vi "CloseEthernetIP connection.vi"(8 "error in (no error)":errorcluster, 11 ".NET Refnum in":refnum<k24>) -> (0 "error out":errorcluster)   [LabVIEW 2022 SP3, in "Motor Controller.lvclass"]
uses:
  Motor Controller.lvclass
  C:/projects/Digilens_IPLC/Classes/Motor Controller/EEIP.dll
  EEIP.dll
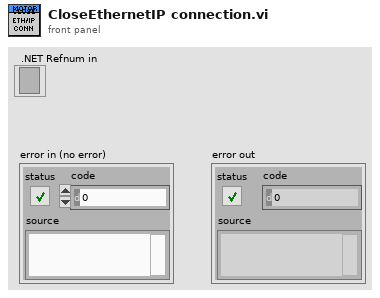
[diagram p1: front panel]
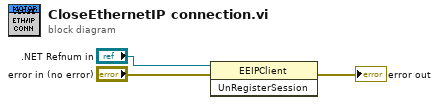
[diagram p0: block diagram]
diagram:
  n1 = invoke class="EEIPClient" method="UnRegisterSession"(reference=".NET Refnum in", error in="error in (no error)") -> (error out=→"error out":errorcluster)  [unwired: 1 in, 2 out]
